vi "conversions (SubVI).vi"(4 "K0":dbl, 5 "Array":dbl[](array[numeric]), 6 "Offset":dbl, 9 "Gain":dbl, 10 "K1":dbl, 11 "RH/T Sensor VSS (V)":dbl) -> (1 "T":dbl, 2 "RH":dbl, 3 "Ethanol":dbl)   [LabVIEW 2014]
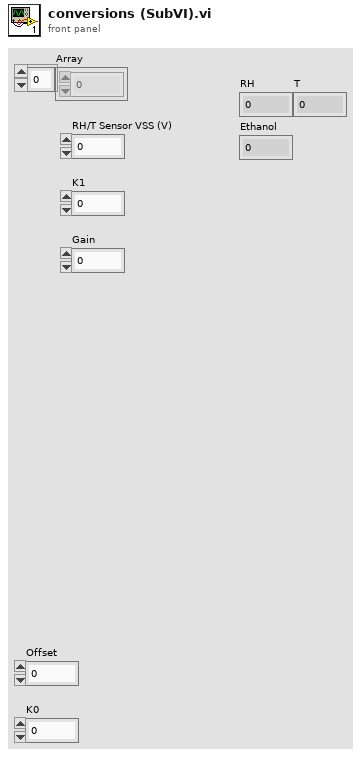
[diagram p1: front panel]
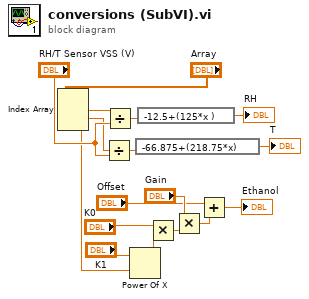
[diagram p0: block diagram]
diagram:
  n1 = Index Array(array="Array") -> (element #1=w5:dbl, element #2=w6:dbl, element #3=w16:dbl)  [unwired: 3 in]
  n2 = Divide(x=w6, y="RH/T Sensor VSS (V)") -> (x/y=w8:dbl)
  n3 = Divide(x=w5, y="RH/T Sensor VSS (V)") -> (x/y=w7:dbl)
  n4 = Power Of X(1:w16, 2:"K1") -> (0:w15:dbl)
  n5 = expression code="-66.875+(218.75*x)"(w8) -> (→"T":dbl)
  n6 = expression code="-12.5+(125*x )"(w7) -> (→"RH":dbl)
  n7 = Multiply(x="K0", y=w15) -> (x*y=w14:dbl)
  n8 = Multiply(x="Gain", y=w14) -> (x*y=w13:dbl)
  n9 = Add(x="Offset", y=w13) -> (x+y=→"Ethanol":dbl)
